vi "Read Short Name.vi"(8 "error in (no error)":errorcluster, 11 "Generic Item in":refnum<class "Generic Item.lvclass">) -> (0 "error out":errorcluster, 2 "Short Name":string, 3 "Generic Item out":refnum<class "Generic Item.lvclass">)   [LabVIEW 2015, in "Item Actor.lvlib" / "Generic Item.lvclass"]
uses:
  Generic Item.lvclass
  Generic Item.lvclass/Generic Item.ctl
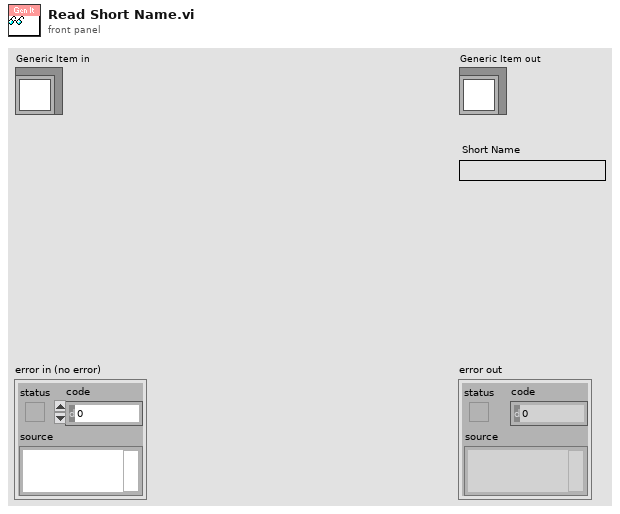
[diagram p1: front panel]
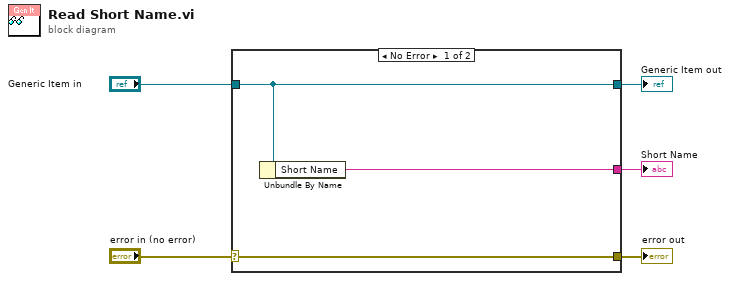
[diagram p0: block diagram]
diagram:
  n1 = case shown="No Error" "error in (no error)" {
    selector: "error in (no error)" -> [w8 w9]
    tunnel: [w8 w9] -> w4
    tunnel: [w7 w10] -> w2
    tunnel: "Generic Item in" -> [w7 w10]
    tunnel: [w6 _] -> w1
    frame No Error {
      n2 = Unbundle By Name(w7) -> ("Short Name"=w6:string)
    }
    frame Error {
    }
  }
  "error out" <- w4
  "Generic Item out" <- w2
  "Short Name" <- w1
